vi "Stop Core.vi"(10 "final error code":i32, 11 "TCP_serverGUI in":refnum<class "TCP_serverGUI.lvclass">) -> (3 "TCP_serverGUI out":refnum<class "TCP_serverGUI.lvclass">)   [LabVIEW 2023, in "TCP_serverGUI.lvlib" / "TCP_serverGUI.lvclass"]
doc: "(<B>Filename</B>: Actor Framework.lvlib:Actor.lvclass:Stop Core.vi)\n\nDefines what the actor does before it stops. Use the <B>final error code</B> input to determine whether the actor shut down in response to an error.\n\nBy default, this method passes the Stop message along to all auto-stop nested actors. A descendant class may override this method to define additional behavior, such as shutting down any processes the actor initiated in its override of the Actor Core method."
uses:
  TCP_serverGUI.lvclass
  TCP_serverGUI.lvclass/TCP_serverGUI.ctl
  <vilib>/ActorFramework/Actor/Actor.lvclass
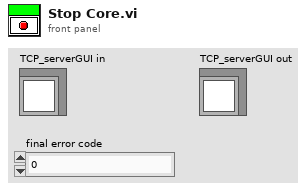
[diagram p1: front panel]
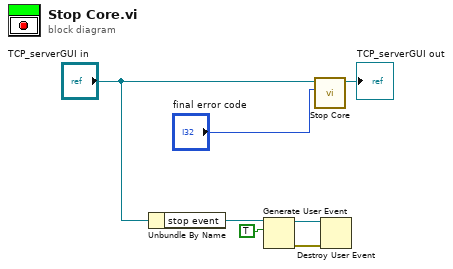
[diagram p0: block diagram]
diagram:
  n1 = Unbundle By Name("TCP_serverGUI in") -> ("stop event"=w4:refnum<user-event>)
  n2 = Generate User Event(user event=w4, event data cluster=TRUE ("event data")) -> (user event out=w2:refnum<user-event>, error out=w1:errorcluster)  [unwired: 2 in]
  n3 = call-parent "Stop Core.vi"("final error code"="final error code", "Actor in"="TCP_serverGUI in") -> ("Actor out"=→"TCP_serverGUI out":refnum<class "TCP_serverGUI.lvclass">)  [unwired: 9 in]
  n4 = Destroy User Event(user event=w2, error in=w1) -> ()  [unwired: 1 out]
